vi "F Dwf Analog In Trigger Length Get.vi"(8 "error in (no error)":errorcluster, 10 "psecLength":dbl, 11 "hdwf":i32) -> (0 "error out":errorcluster, 2 "psecLength out":dbl, 3 "function return":i32)   [LabVIEW 2019, in "Olasdwf.lvlib"]
doc: "DWFAPI int FDwfAnalogInTriggerLengthGet(HDWF hdwf, double *psecLength);"
uses:
  Olasdwf.lvlib
  Windows/System32/dwf.dll
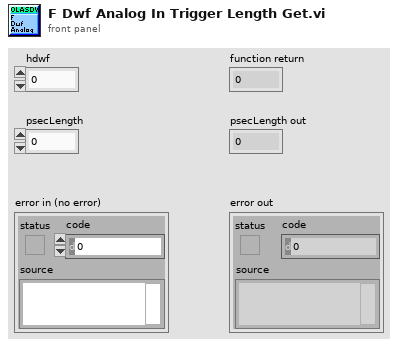
[diagram p1: front panel]
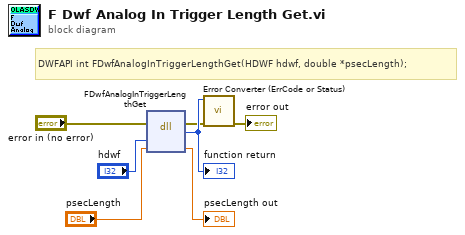
[diagram p0: block diagram]
diagram:
  # "DWFAPI int FDwfAnalogInTriggerLengthGet(HDWF hdwf, double *psecLength);"
  n1 = dll-call lib="C:/Windows/System32/dwf.*" fn="FDwfAnalogInTriggerLengthGet"(error in="error in (no error)", "hdwf"="hdwf", "psecLength"="psecLength") -> (error out=w2:errorcluster, w7:i32, "psecLength"=→"psecLength out":dbl)  [unwired: 3 in, 1 out]
  "function return" <- w7
  n2 = call "Error Converter (ErrCode or Status).vi"("error in (no error)"=w2, "error code"=w7) -> ("error out"=→"error out":errorcluster)  [unwired: 9 in]
